vi "Distort Image (Greyscale).vi"(5 "Border Type (Default: Constant)":T1, 6 "Use Fixed Point Remapping (Default: False)":bool, 7 "Value (Default: 0)":u8, 8 "error in (no error)":errorcluster, 9 "Greyscale Image Destination in":T2, 10 "Greyscale Image Source in":T2, 11 "Image Distorter in":refnum<class "Image Distorter.lvclass">) -> (0 "error out":errorcluster, 2 "Greyscale Image Destination":T2, 3 "Image Distorter":refnum<class "Image Distorter.lvclass">)   [LabVIEW 2020, in "image.lvlib" / "Image Distorter.lvclass"]
doc: "Apply distortion to the Source Image."
uses:
  Image Distorter.lvclass
  Greyscale Image.ctl
  Border Type.ctl
  Image Distorter.lvclass/Image Distorter.ctl
  ccc224f2-fea8-4097-85c8-c2b3fe04188f.vi
  <vilib>/Utility/error.llb/Error Cluster From Error Code.vi
  image.lvlib
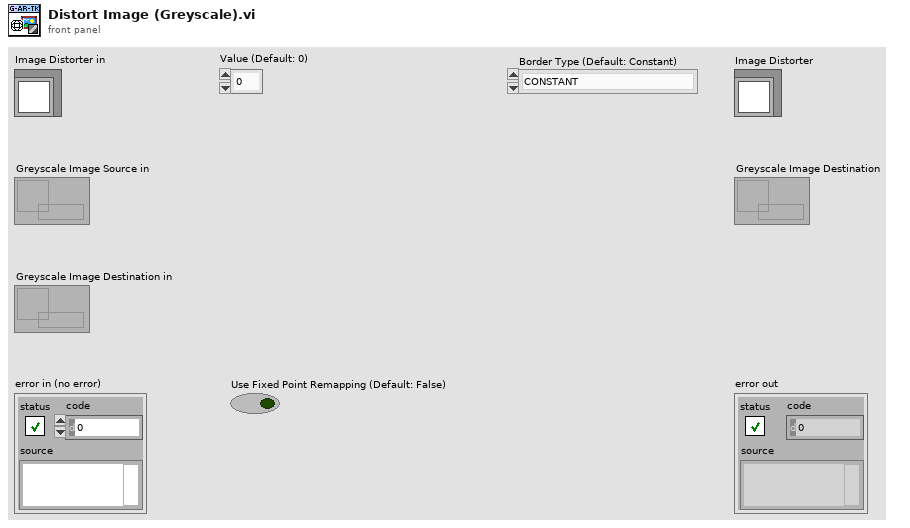
[diagram p1: front panel]
types:
  T1 = typedef "image.lvlib/Border Type.ctl" = enum8{"CONSTANT", "REPLICATE", "REFLECT", "WRAP", "TRANSPARENT", "DEFAULT", "ISOLATED"}
  T2 = typedef "image.lvlib/Greyscale Image.ctl" = refnum<data-value>
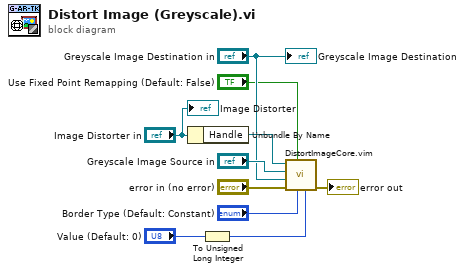
[diagram p0: block diagram]
diagram:
  n1 = Unbundle By Name("Image Distorter in") -> ("Handle"=w9:refnum<data-value>)
  n2 = To Unsigned Long Integer(number="Value (Default: 0)") -> (unsigned 32bit integer=w2:u32)
  n3 = call "DistortImageCore.vim"("Colour"=w2, "Border Type"="Border Type (Default: Constant)", "Use Fixed Point remapping"="Use Fixed Point Remapping (Default: False)", "error in (no error)"="error in (no error)", "Destination Image"="Greyscale Image Destination in", "Source Image"="Greyscale Image Source in", "Handle"=w9) -> ("error out"=→"error out":errorcluster)  [unwired: 4 in]
  "Image Distorter" <- "Image Distorter in"
  "Greyscale Image Destination" <- "Greyscale Image Destination in"
